vi "vna preset.vi"(8 "error in (no error)":errorcluster, 11 "VISA resource name":refnum<visa-resource-name>) -> (0 "error out":errorcluster, 3 "VISA resource name 2":refnum<visa-resource-name>)   [LabVIEW 2013]
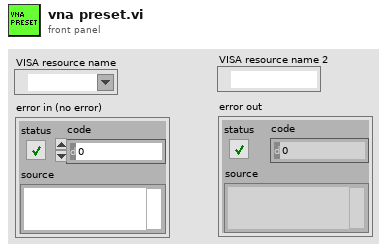
[diagram p1: front panel]
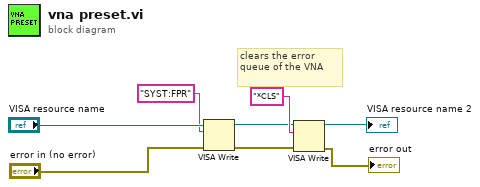
[diagram p0: block diagram]
diagram:
  # "clears the error queue of the VNA"
  n1 = VISA Write(VISA resource name="VISA resource name", write buffer="SYST:FPR", error in (no error)="error in (no error)") -> (VISA resource name out=w4:refnum<visa-resource-name>, error out=w3:errorcluster)  [unwired: 1 out]
  n2 = VISA Write(VISA resource name=w4, write buffer="*CLS", error in (no error)=w3) -> (VISA resource name out=→"VISA resource name 2":refnum<visa-resource-name>, error out=→"error out":errorcluster)  [unwired: 1 out]
